vi "Calculate_Timescales.vi"(1 "Sampling Frequency (Hz)":dbl, 2 "Autocorrelation length":i32, 3 "Autocorrelation":dbl[](array[numeric])) -> (0 "Time Scale estimate (s)":dbl)   [LabVIEW 2010]
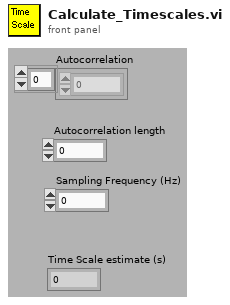
[diagram p1: front panel]
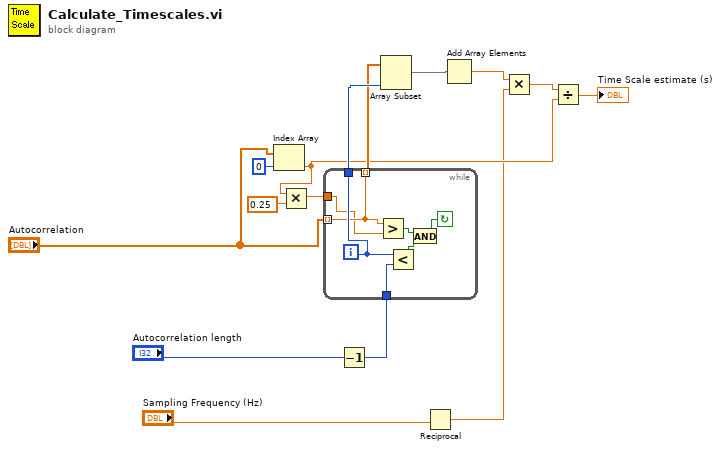
[diagram p0: block diagram]
diagram:
  n1 = Index Array(array="Autocorrelation", index=0) -> (element=w4:dbl)
  n2 = Multiply(x=w4, y=0.25) -> (x*y=w15:dbl)
  n3 = Decrement(x="Autocorrelation length") -> (x-1=w8:i32)
  n4 = while {
    tunnel: "Autocorrelation" -> [w18] mode=indexing
    tunnel: w8 -> [w22]
    tunnel: [w18] -> w11 mode=indexing
    tunnel: [w19] -> w12
    tunnel: w15 -> [w17]
    i -> [w19]
    stop <- w20 continue-if-true
    n5 = Greater?(x=w18, y=w17) -> (0:w16:bool)
    n6 = Less?(x=w19, y=w22) -> (x < y?=w21:bool)
    n7 = And(x=w16, y=w21) -> (x .and. y?=w20:bool)
  }
  n8 = Array Subset(array=w11, length=w12) -> (w7:dbl[])  [unwired: 1 in]
  n9 = Reciprocal(x="Sampling Frequency (Hz)") -> (1/x=w3:dbl)
  n10 = Add Array Elements(numeric array=w7) -> (sum=w6:dbl)
  n11 = Multiply(x=w6, y=w3) -> (x*y=w5:dbl)
  n12 = Divide(x=w5, y=w4) -> (x/y=→"Time Scale estimate (s)":dbl)
